vi "Front Panel Visual.vi"() -> ()   [LabVIEW 2009]
panel:
  in  "Power":bool
  out "Motor Controller":bool
  out "Cameras":bool
  out "SICK":bool
  out "GPS":bool
  out "Compass":bool
  out "Communication":bool
  out "Compact RIO":bool
  out "EVS":bool
  in  "Safety":bool
  in  "Initialize":bool
  in  "GO":bool
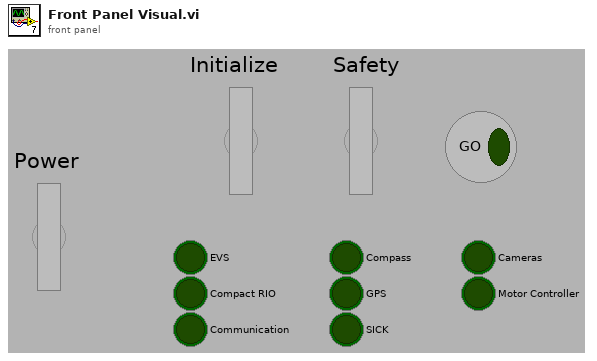
[diagram p1: front panel]
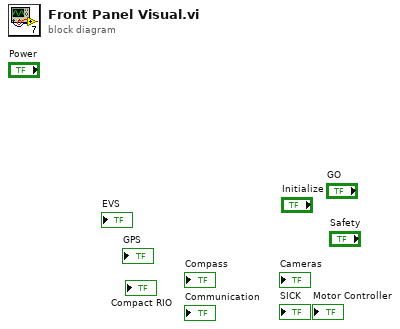
[diagram p0: block diagram]
diagram:
